vi "RemoveChecksum.vi"(4 "IN":string) -> (0 "Check OK?":bool, 1 "OUT":string)   [LabVIEW 2014]
doc: "Remove checksom from file content and chech it's value"
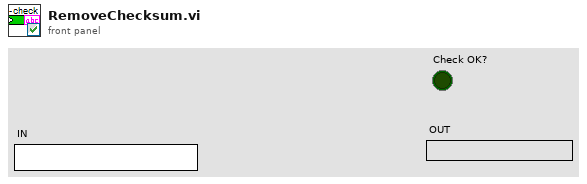
[diagram p1: front panel]
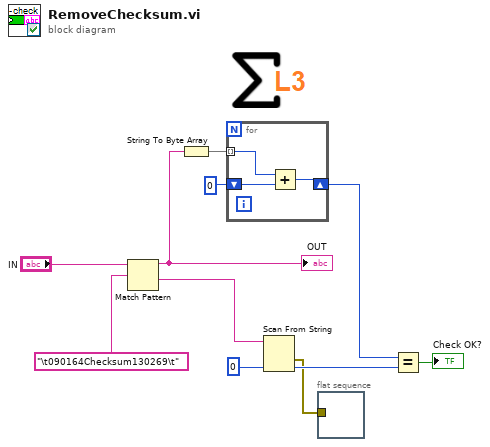
[diagram p0: block diagram]
diagram:
  n1 = Match Pattern(string="IN", regular expression="\t090164Checksum130269\t" ("format string")) -> (before substring=w6:string, after substring=w9:string)  [unwired: 1 in, 2 out]
  "OUT" <- w6
  n2 = String To Byte Array(string=w6) -> (unsigned byte array=w8:u8[])
  n3 = for {
    tunnel: w8 -> [w13] mode=indexing
    shift-right: [w12] -> w3
    shift-left: u64 0 -> [w14]
    n4 = Add(x=w13, y=w14) -> (x+y=w12:u64)
  }
  n5 = Scan From String(input string=w9, default 1=u64 0) -> (error out=w1:errorcluster, output 1=w4:u64)  [unwired: 3 in, 2 out]
  n6 = flat-sequence {
    tunnel: w1 -> [_]
    frame #0 {
    }
  }
  n7 = Equal?(x=w3, y=w4) -> (x = y?=→"Check OK?":bool)
